vi "MALT CardReqCreate.vi"(7 "Cmd":string, 8 "error in":errorcluster, 9 "Port":i32, 10 "Address":i32, 11 "CardType":T1=enum."MALT132") -> (0 "error out":errorcluster, 3 "request":string)   [LabVIEW 2018]
uses:
  Types/MALT CardTypes.ctl
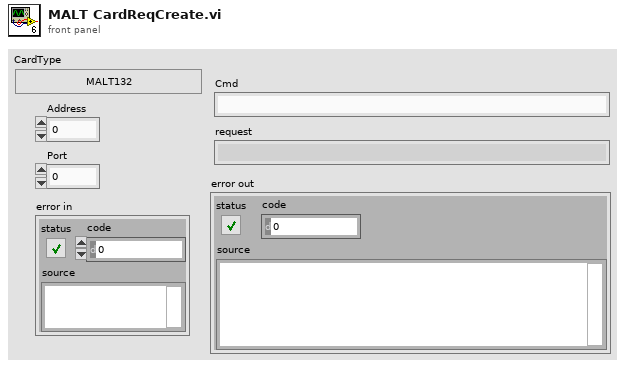
[diagram p1: front panel]
types:
  T1 = typedef "MALT CardTypes.ctl" = enum32{"-", "YAV90832", "YAV904X8", "MALT132", "YAV91616", "YAV90PIN", "YAV90096", "YAV90HVT", "YAV90CLR", "YAV90128", "YAV90PNE", "YAVCANCON", "YAV91775", "YAV90XXX", "YAV90MMU", "H730050", "H710060", "H710061", "YAV90304", "MMI", "YAV90060", "YAV90MUX", "YAV90059", "Not Defined"}
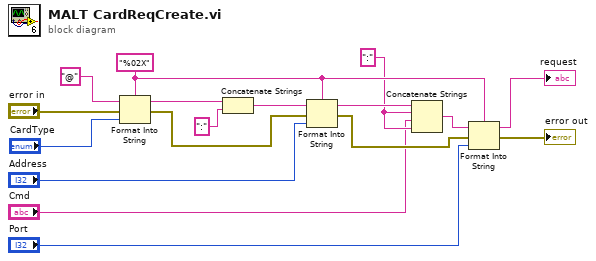
[diagram p0: block diagram]
diagram:
  w4 = ":" ("resulting string")
  w7 = "%02X" ("format string")
  n1 = Format Into String(format string=w7, initial string="@", error in="error in", "CardType") -> (resulting string=w16:string, error out=w11:errorcluster)
  n2 = Concatenate Strings(w16, ":" ("string")) -> (w14:string)
  n3 = Format Into String(format string=w7, initial string=w14, error in=w11, "Address") -> (resulting string=w12:string, error out=w9:errorcluster)
  n4 = Concatenate Strings(w12, w4, "Cmd", w4) -> (w10:string)
  n5 = Format Into String(format string=w7, initial string=w10, error in=w9, "Port") -> (resulting string=→"request":string, error out=→"error out":errorcluster)
